vi "HEART_BEAT.vi"(8 "error in (no error)":errorcluster, 11 "Message":T1={"Payload Size"=0, "Sequence Number"=0, "Sensor Type"=enum."APP", "Message Types"=enum."SEND_LOG_FILE_SIZE", "Data"=[]}) -> (0 "error out":errorcluster, 3 "HB Good?":bool)   [LabVIEW 2019]
uses:
  Typedefs/Sensor Types.ctl
  Typedefs/Message Types.ctl
  Typedefs/Message.ctl
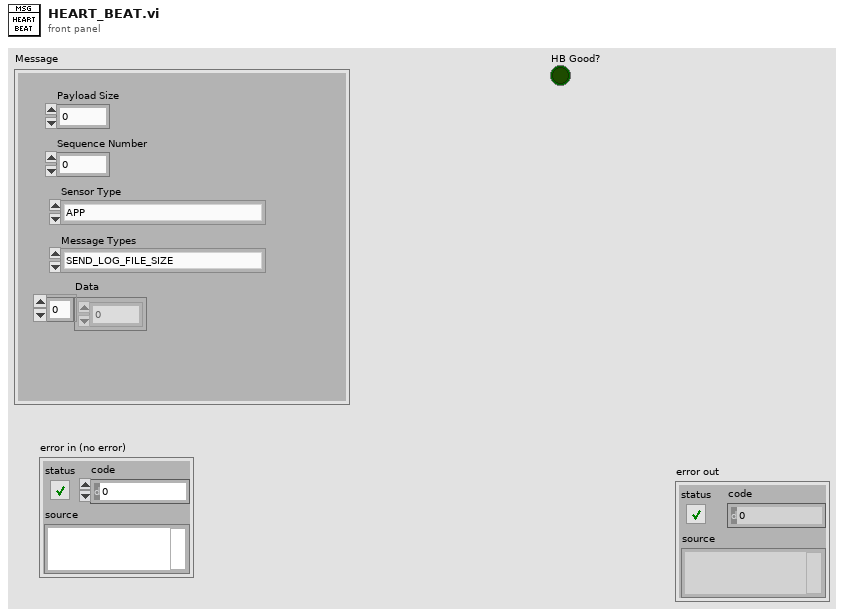
[diagram p1: front panel]
types:
  T1 = typedef "Message.ctl" = cluster{"Payload Size":u8, "Sequence Number":u8, "Sensor Type":T2, "Message Types":T3, "Data":u8[]}
  T2 = typedef "Sensor Types.ctl" = enum16{"APP", "TURBIDITY", "PH"}
  T3 = typedef "Message Types.ctl" = enum16{"HEART_BEAT", "CONNECT", "GET_CURRENT_MEASUREMENTS", "GET_LOG_FILE", "SEND_LOG_FILE_SIZE", "SEND_LOG_FILE_CHUNK", "GET_LOGGING_PERIOD", "SET_LOGGING_PERIOD", "SEND_SD_CARD_INFO", "GET_LOGS_LIST", "SEND_LOG_FILE_NAME", "SEND_LOGGING_PERIOD", "GET_RTC_TIME", "SET_RTC_TIME", "SEND_RTC_TIME", "SEND_CURRENT_MEASUREMENTS", "DELETE_LOG_FILE", "GET_SD_CARD_INFO", "GET_BATTERY_INFO", "SEND_BATTERY_INFO", "GET_LOG_FILE_SIZE", "ERROR_MSG"}
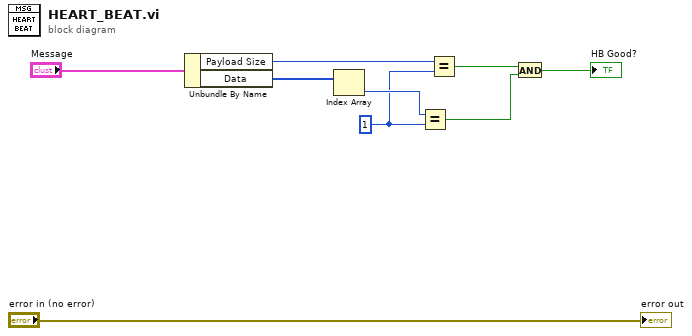
[diagram p0: block diagram]
diagram:
  w4 = u8 1 ("y")
  n1 = Unbundle By Name("Message") -> ("Payload Size"=w5:u8, "Data"=w8:u8[])
  n2 = Index Array(array=w8) -> (element=w7:u8)  [unwired: 1 in]
  n3 = Equal?(x=w7, y=w4) -> (x = y?=w2:bool)
  n4 = Equal?(x=w5, y=w4) -> (x = y?=w3:bool)
  n5 = And(x=w3, y=w2) -> (x .and. y?=→"HB Good?":bool)
  "error out" <- "error in (no error)"
